vi "FrecAmpGEN.vi"(8 "error in (no error)":errorcluster, 9 "Frec (Hz)":dbl, 10 "Amplitud (Vrms)":dbl) -> (0 "error out":errorcluster)   [LabVIEW 2019, in "DS360_GPIB.lvlib"]
uses:
  DS360_GPIB.lvlib
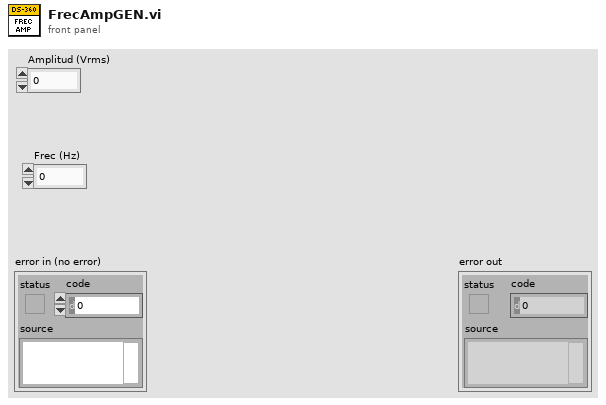
[diagram p1: front panel]
types:
  T1 = cluster{"error":bool, "code":i32, "source":string}
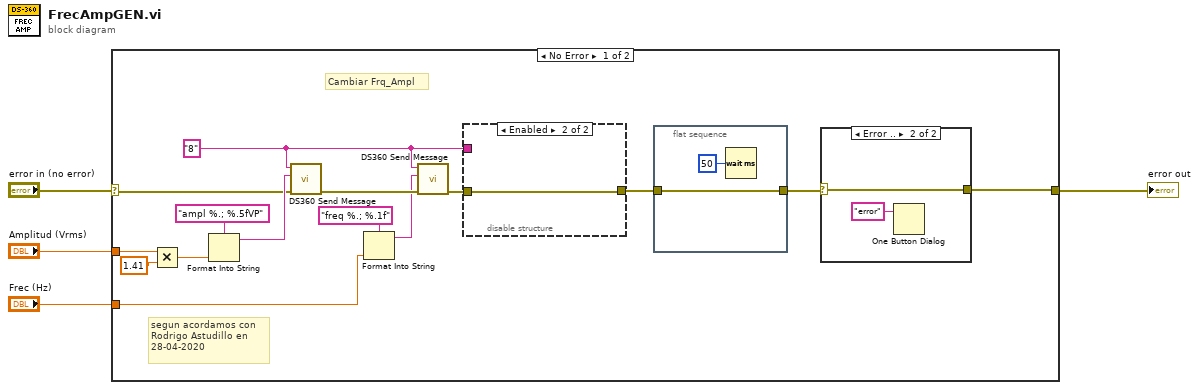
[diagram p0: block diagram]
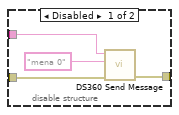
[diagram p3: hidden frame]
diagram:
  n1 = case shown="No Error" "error in (no error)" {
    selector: "error in (no error)" -> [w12 w30]
    tunnel: [w5 w30] -> w3
    tunnel: "Amplitud (Vrms)" -> [w10 _]
    tunnel: "Frec (Hz)" -> [w11 _]
    frame No Error {
      w13 = "8" ("write buffer")
      # "segun acordamos con\nRodrigo Astudillo en\n28-04-2020"
      # "Cambiar Frq_Ampl"
      n2 = Multiply(x=w10, y=1.41) -> (x*y=w8:dbl)
      n3 = Format Into String(format string="ampl %.; %.5fVP" ("write buffer"), w8) -> (resulting string=w16:string)  [unwired: 2 in, 1 out]
      n4 = call <instrlib>:"DS360 Send Message.vi"("address string"=w13, "write buffer"=w16, "error in"=w12) -> ("error out"=w19:T1)  [unwired: 3 in, 3 out]
      n5 = Format Into String(format string="freq %.; %.1f" ("write buffer"), w11) -> (resulting string=w14:string)  [unwired: 2 in, 1 out]
      n6 = call <instrlib>:"DS360 Send Message.vi"("address string"=w13, "write buffer"=w14, "error in"=w19) -> ("error out"=w18:T1)  [unwired: 3 in, 3 out]
      n7 = disable-structure shown="Enabled" {
        disable-tunnel: w18 -> [w27 w29]
        disable-tunnel: w13 -> [w26 _]
        disable-tunnel: [w25 w29] -> w7
        frame Disabled {
          n8 = call <instrlib>:"DS360 Send Message.vi"("address string"=w26, "write buffer"="mena 0", "error in"=w27) -> ("error out"=w25:T1)  [unwired: 3 in, 3 out]
        }
        frame Enabled {
        }
      }
      n9 = flat-sequence {
        tunnel: w7 -> [w23]
        tunnel: [w23] -> w6
        frame #0 {
          n10 = Wait (ms)(milliseconds to wait=u32 50) -> ()  [unwired: 1 out]
        }
      }
      n11 = case shown="Error .." w6 {
        selector: w6 -> [w20 w22]
        tunnel: [w20 w22] -> w5
        frame No Error {
        }
        frame Error {
          n12 = One Button Dialog(message="error") -> ()  [unwired: 1 in, 1 out]
        }
      }
    }
    frame Error {
    }
  }
  "error out" <- w3
